vi "overaly grid numbers.vi"(4 "Circles":cluster{"x":dbl, "y":dbl, "r":dbl}[](array[cluster]), 5 "y":dbl[](array[numeric]), 6 "x":dbl[](array[numeric]), 7 "Refnum in":T1) -> (0 "cy":dbl[](array[numeric]), 1 "cx":dbl[](array[numeric]), 2 "Circles 2":cluster{"x":dbl, "y":dbl, "r":dbl}[](array[cluster]), 3 "Refnum out":T1)   [LabVIEW 2018]
uses:
  <vilib>/vision/Image Controls.llb/IMAQ Image.ctl
panel:
  in  "step":dbl
  in  "Y0":dbl
  in  "X0":dbl
  in  "nY":i8
  in  "nX":i8
  out "X":i32[](array[numeric])
  out "Y":i32[](array[numeric])
  out "max x":dbl
  out "min x":dbl
  out "max y":dbl
  out "min y":dbl
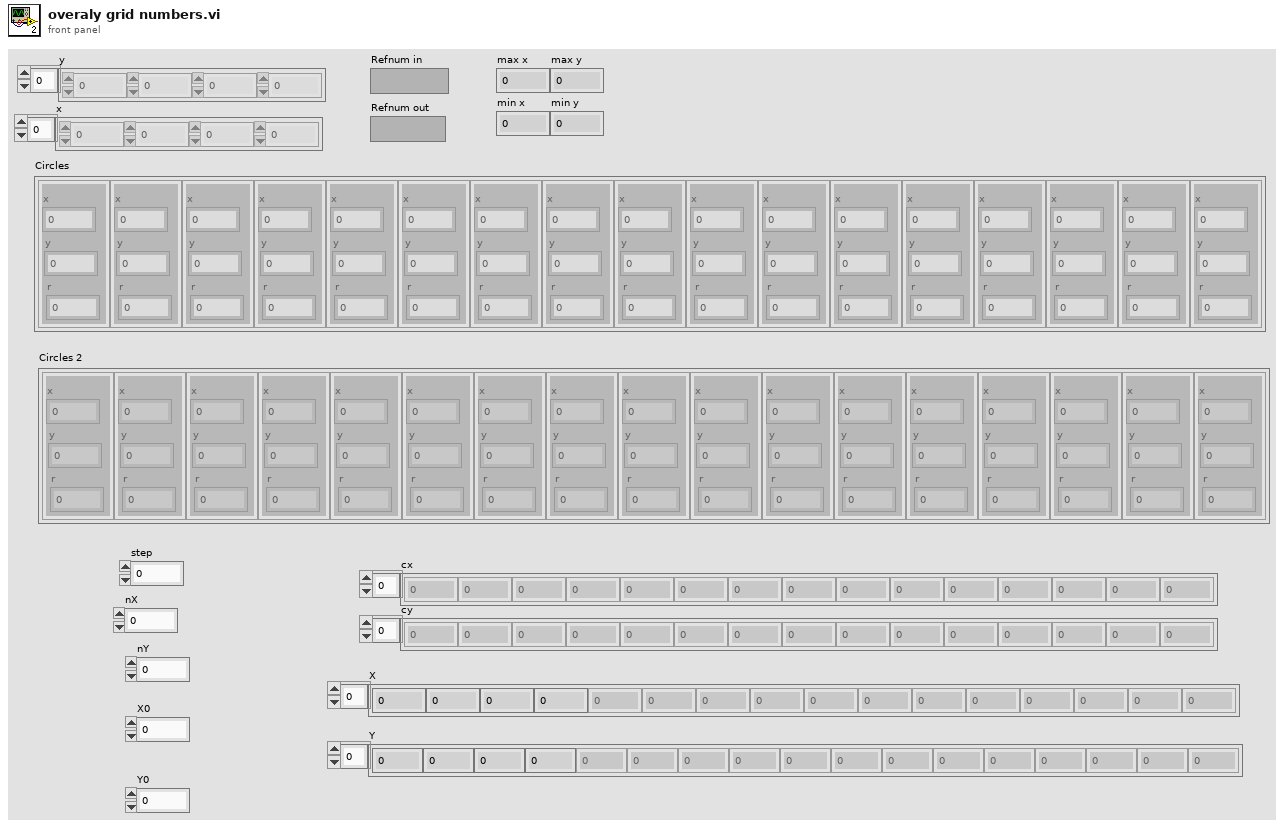
[diagram p1: front panel]
types:
  T1 = typedef "IMAQ Image.ctl" = refnum<image>
  T2 = cluster{"Desired Font (Application)":enum16{"User-specified Font", "Application Font", "System Font", "Dialog Font"}, "[User-specified Font]":cluster{"Font Name":string, "Size":i16, "Strikeout?":bool, "Italic?":bool, "Underline?":bool, "Outline?":bool, "Shadow?":bool, "Bold?":bool, "Rotation Angle":dbl}, "Horizontal Alignment":i16, "Vertical Alignment":i16}
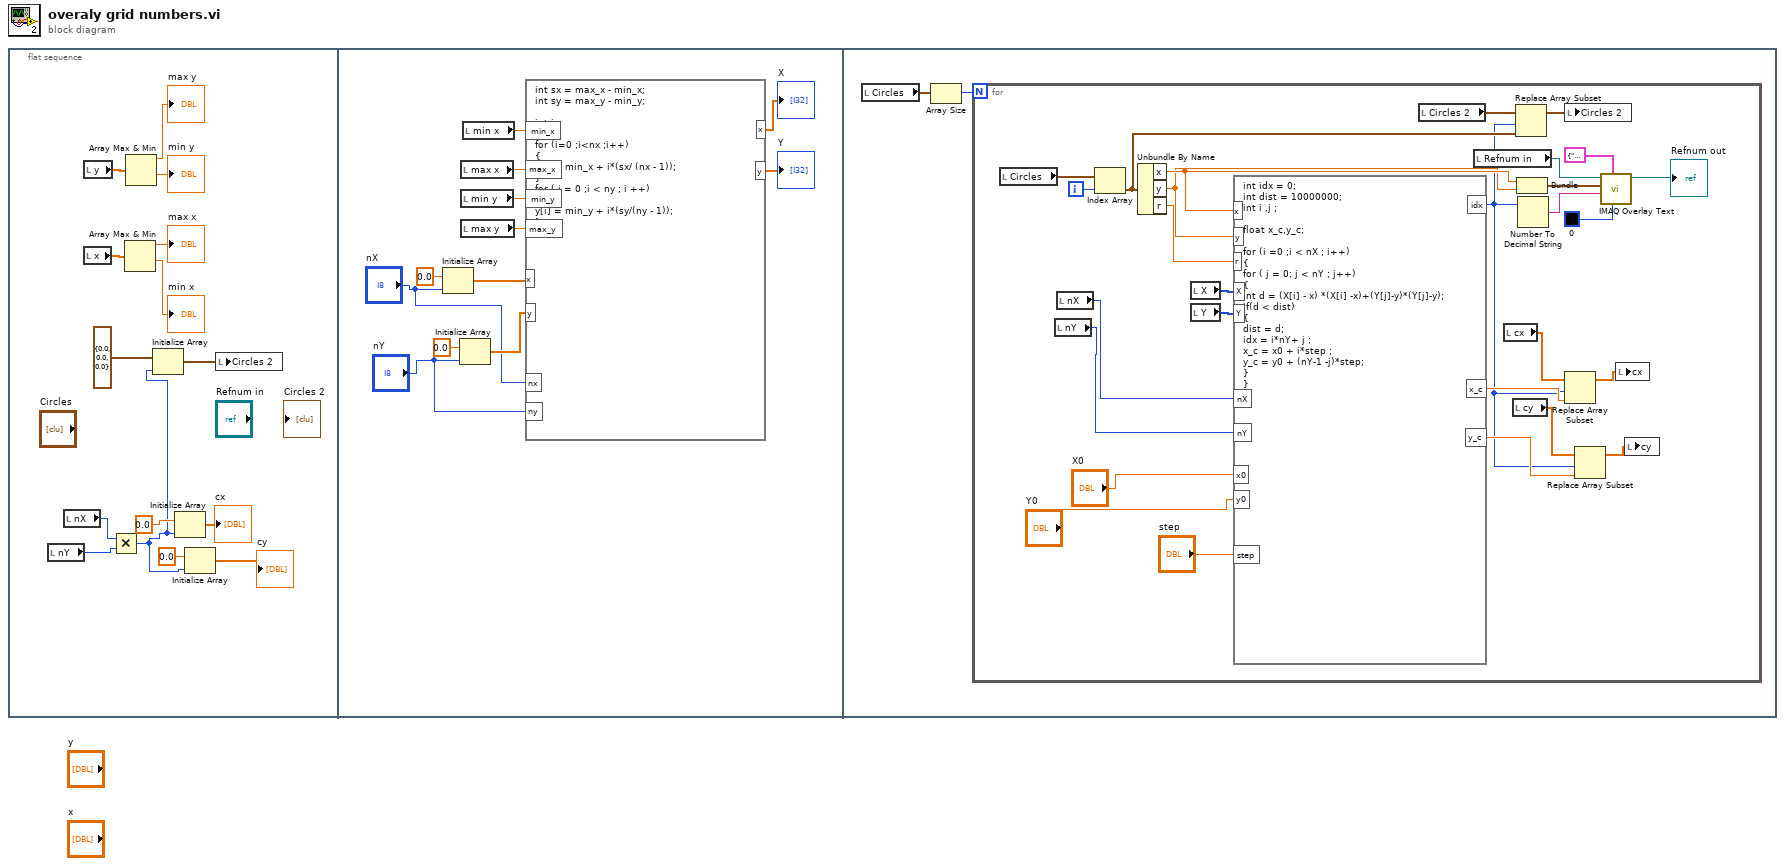
[diagram p0: block diagram]
diagram:
  n1 = flat-sequence {
    frame #0 {
      n2 = local read "nY"() -> (w2:i8)
      n3 = local read "nX"() -> (w3:i8)
      n4 = local read "y"() -> (w14:dbl[])
      n5 = local read "x"() -> (w15:dbl[])
      n6 = Multiply(x=w3, y=w2) -> (x*y=w1:i8)
      n7 = Array Max & Min(array=w15) -> (max value=→"max x":dbl, min value=→"min x":dbl)  [unwired: 2 out]
      n8 = Array Max & Min(array=w14) -> (max value=→"max y":dbl, min value=→"min y":dbl)  [unwired: 2 out]
      n9 = Initialize Array(cluster{"x":dbl, "y":dbl, "r":dbl} {"x"=0.0, "y"=0.0, "r"=0.0} ("circle"), w1) -> (w9:cluster{"x":dbl, "y":dbl, "r":dbl}[])
      n10 = Initialize Array(0.0 ("element"), w1) -> (→"cx":dbl[])
      n11 = Initialize Array(0.0 ("element"), w1) -> (→"cy":dbl[])
      n12 = local write "Circles 2"(w9) -> ()
    }
    frame #1 {
      n13 = Initialize Array(0.0 ("element"), "nX") -> (w21:dbl[])
      n14 = Initialize Array(0.0 ("element"), "nY") -> (w18:dbl[])
      n15 = local read "max x"() -> (w26:dbl)
      n16 = local read "min y"() -> (w25:dbl)
      n17 = local read "max y"() -> (w24:dbl)
      n18 = local read "min x"() -> (w27:dbl)
      n19 = formula code="int sx = max_x - min_x;\nint sy = max_y - min_y;\n\nint i;\nint j;\nfor (i=0 ;i<nx ;i++)\n{\nx[i] = min_x + i*(sx/ (nx - 1));\n}\nfor ( i = 0 ;i < ny ; i ++)\n{\ny[i] = min_y + i*(sy/(ny - 1));\n}"("min_x"=w27, "max_x"=w26, "min_y"=w25, "max_y"=w24, "x"=w21, "y"=w18, "nx"="nX", "ny"="nY") -> ("x"=→"X":dbl[], "y"=→"Y":dbl[])
    }
    frame #2 {
      n20 = local read "Circles"() -> (w28:cluster{"x":dbl, "y":dbl, "r":dbl}[])
      n21 = Array Size(array=w28) -> (size(s)=w29:i32)
      n22 = for {
        N: w29 -> [_]
        i -> [w51]
        n23 = local read "Circles"() -> (w57:cluster{"x":dbl, "y":dbl, "r":dbl}[])
        n24 = local read "nY"() -> (w39:i8)
        n25 = local read "nX"() -> (w38:i8)
        n26 = Index Array(array=w57, index=w51) -> (element=w50:cluster{"x":dbl, "y":dbl, "r":dbl})
        n27 = Unbundle By Name(w50) -> ("x"=w48:dbl, "y"=w47:dbl, "r"=w54:dbl)
        n28 = local read "X"() -> (w56:i32[])
        n29 = local read "Y"() -> (w55:i32[])
        n30 = formula code="int idx = 0;\nint dist = 10000000;\nint i ,j ;\n\nfloat x_c,y_c;\n\nfor (i =0 ;i < nX ; i++)\n{\nfor ( j = 0; j < nY ; j++)\n{\nint d = (X[i] - x) *(X[i] -x)+(Y[j]-y)*(Y[j]-y);\nif(d < dist) \n{\ndist = d;\nidx = i*nY+ j ;\nx_c = x0 + i*step ;\ny_c = y0 + (nY-1 -j)*step;\n}\n}\n}"("x"=w48, "y"=w47, "r"=w54, "X"=w56, "Y"=w55, "nX"=w38, "nY"=w39, "x0"="X0", "y0"="Y0", "step"="step") -> ("idx"=w30:i32, "x_c"=w32:dbl, "y_c"=w31:dbl)
        n31 = local read "Circles 2"() -> (w52:cluster{"x":dbl, "y":dbl, "r":dbl}[])
        n32 = local read "Refnum in"() -> (w43:T1)
        n33 = local read "cx"() -> (w36:dbl[])
        n34 = local read "cy"() -> (w34:dbl[])
        n35 = Replace Array Subset(array=w52, new element=w50, index=w30) -> (w53:cluster{"x":dbl, "y":dbl, "r":dbl}[])
        n36 = Bundle("x"=w48, "y"=w47) -> (w49:cluster{"x":dbl, "y":dbl})  [unwired: 1 in]
        n37 = Number To Decimal String(number=w30) -> (decimal integer string=w46:string)  [unwired: 1 in]
        n38 = local write "Circles 2"(w53) -> ()
        n39 = Replace Array Subset(array=w36, new element=w32, index=w30) -> (w35:dbl[])
        n40 = Replace Array Subset(array=w34, new element=w31, index=w30) -> (w33:dbl[])
        n41 = call "IMAQ Overlay Text"("Text Color (black)"=u32 0, "Font, Size & Style"=T2 {"Desired Font (Application)"=enum."User-specified Font", "[User-specified Font]"={"Font Name"="", "Size"=25, "Strikeout?"=FALSE, "Italic?"=FALSE, "Underline?"=TRUE, "Outline?"=FALSE, "Shadow?"=TRUE, "Bold?"=TRUE, "Rotation Angle"=0.0}, "Horizontal Alignment"=1, "Vertical Alignment"=2}, "String"=w46, "Origin"=w49, "Image"=w43) -> ("Image Out"=→"Refnum out":T1)  [unwired: 5 in, 1 out]
        n42 = local write "cx"(w35) -> ()
        n43 = local write "cy"(w33) -> ()
      }
    }
  }
